vi "UEvent_MONITOR_VBAT.vi"(6 "Vout  - Vbat profile":enum16{"3.8VDC", "2.9VDC", "By Pass", "4.0VDC"}(ring), 9 "USB":tag, 10 "Range - Shunts":T1, 11 "Refnum in":refnum<k21>) -> (0 "error out":errorcluster, 1 "DUT_Voltage":dbl, 2 "Battery_Voltage":dbl, 3 "Refnum out":refnum<k21>, 5 "Power ON/OFF":bool, 7 "DevSerialNum":u32)   [LabVIEW 2015]
uses:
  Range_Shunt_selector.ctl
panel:
  in  "error in (no error)":errorcluster
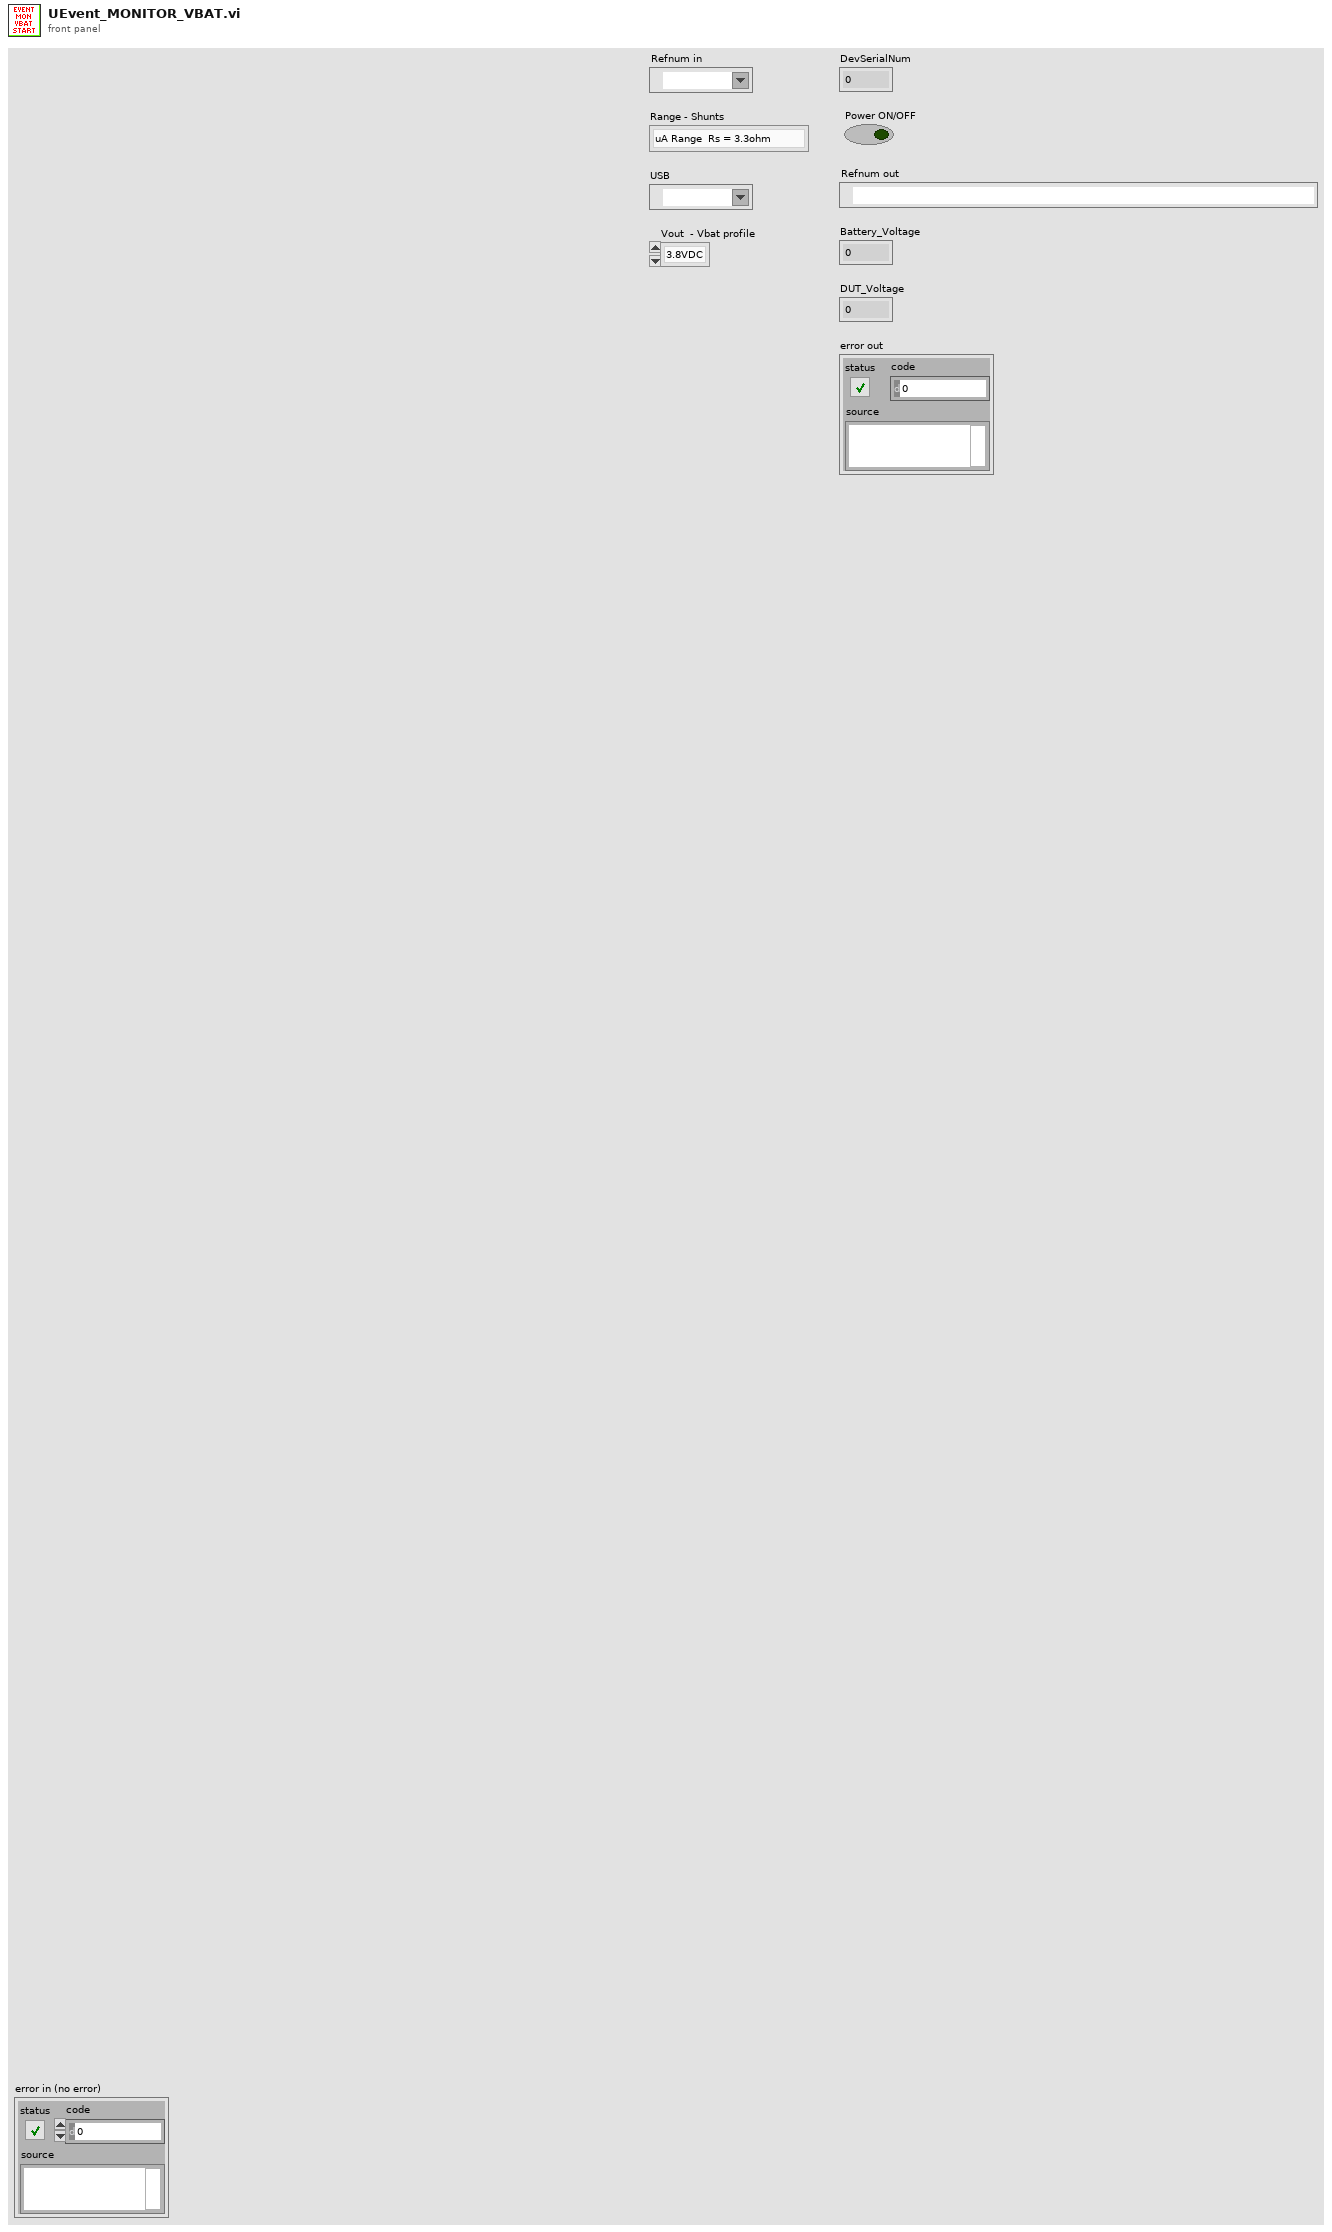
[diagram p1: front panel]
types:
  T1 = typedef "Range_Shunt_selector.ctl" = enum16{"uA Range  Rs = 3.3ohm", "mA Range Rs = 3.3Ohm", "mA Range Rs = 1Ohm", "mA Range Rs = 1Ohm - X2"}
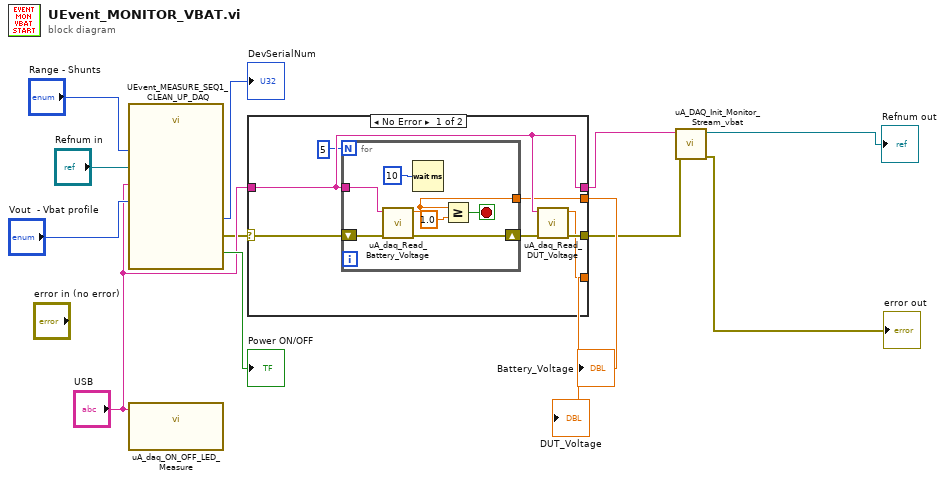
[diagram p0: block diagram]
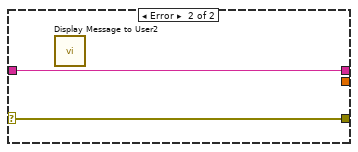
[diagram p2: hidden frame]
diagram:
  n1 = call "UEvent_MEASURE_SEQ1_CLEAN_UP_DAQ.vi"("USB  in"="USB", "Vout  - Vbat profile"="Vout  - Vbat profile", "Range - Shunts in"="Range - Shunts", "TASK IN"="Refnum in") -> ("error out"=w5:errorcluster, "DevSerialNum"=→"DevSerialNum":u32, "Power ON/OFF"=→"Power ON/OFF":bool)  [unwired: 5 in]
  n2 = call "uA_daq_ON_OFF_LED_Measure.vi"("USB"="USB") -> ()  [unwired: 10 in, 1 out]
  n3 = case shown="No Error" w5 {
    selector: w5 -> [w19 w29]
    tunnel: "USB" -> [w17 w28]
    tunnel: [w18 w29] -> w3
    tunnel: [w17 w28] -> w4
    tunnel: [w14 _] -> w6
    tunnel: [w16 _] -> w7
    frame No Error {
      n4 = for {
        N: 5 -> [_]
        tunnel: w17 -> [w25]
        shift-right: [w27] -> w20
        shift-left: w19 -> [w26]
        tunnel: [w23] -> w14
        stop <- w24 stop-if-true
        n5 = call "uA_daq_Read_Battery_Voltage.vi"("error in"=w26, "USB DAQ"=w25) -> ("error out"=w27:errorcluster, "Battery_Voltage"=w23:dbl)  [unwired: 8 in]
        n6 = Wait (ms)(milliseconds to wait=u32 10) -> ()  [unwired: 1 out]
        n7 = Greater Or Equal?(x=w23, y=1.0) -> (x >= y?=w24:bool)
      }
      n8 = call "uA_daq_Read_DUT_Voltage.vi"("error in"=w20, "USB DAQ"=w17) -> ("error out"=w18:errorcluster, "DUT_Voltage"=w16:dbl)  [unwired: 8 in]
    }
    frame Error {
      n9 = call "Display Message to User2"() -> ()  [unwired: 10 in, 2 out]
    }
  }
  "DUT_Voltage" <- w7
  "Battery_Voltage" <- w6
  n10 = call "uA_DAQ_Init_Monitor_Stream_vbat.vi"("error in (no error)"=w3, "USB"=w4) -> ("error out"=→"error out":errorcluster, "Refnum out"=→"Refnum out":refnum<k21>)  [unwired: 8 in]
